vi "TTA_MATLAB_RFICPALLinearizationTest.vi"(0 "Sub-Function Name":string, 1 "Instrument Cluster In":T1, 5 "Test Group":string, 11 "error in":errorcluster) -> (4 "SubTestSuccess":dbl[](array[numeric]), 12 "Instrument Cluster Out":T1, 15 "error out":errorcluster)   [LabVIEW 2016]
uses:
  TTA_Controls/TTA_Control_Complete_Settings_Cluster.ctl
  TTA_Controls/TTA_Control_Instrument_Cluster.ctl
  TTA_Globals/TTA_Global_Complete_Settings.vi
panel:
  out "Test Status":string
  in  "Complete Settings Cluster":T2
  out "RFICs":i32[](array[numeric])
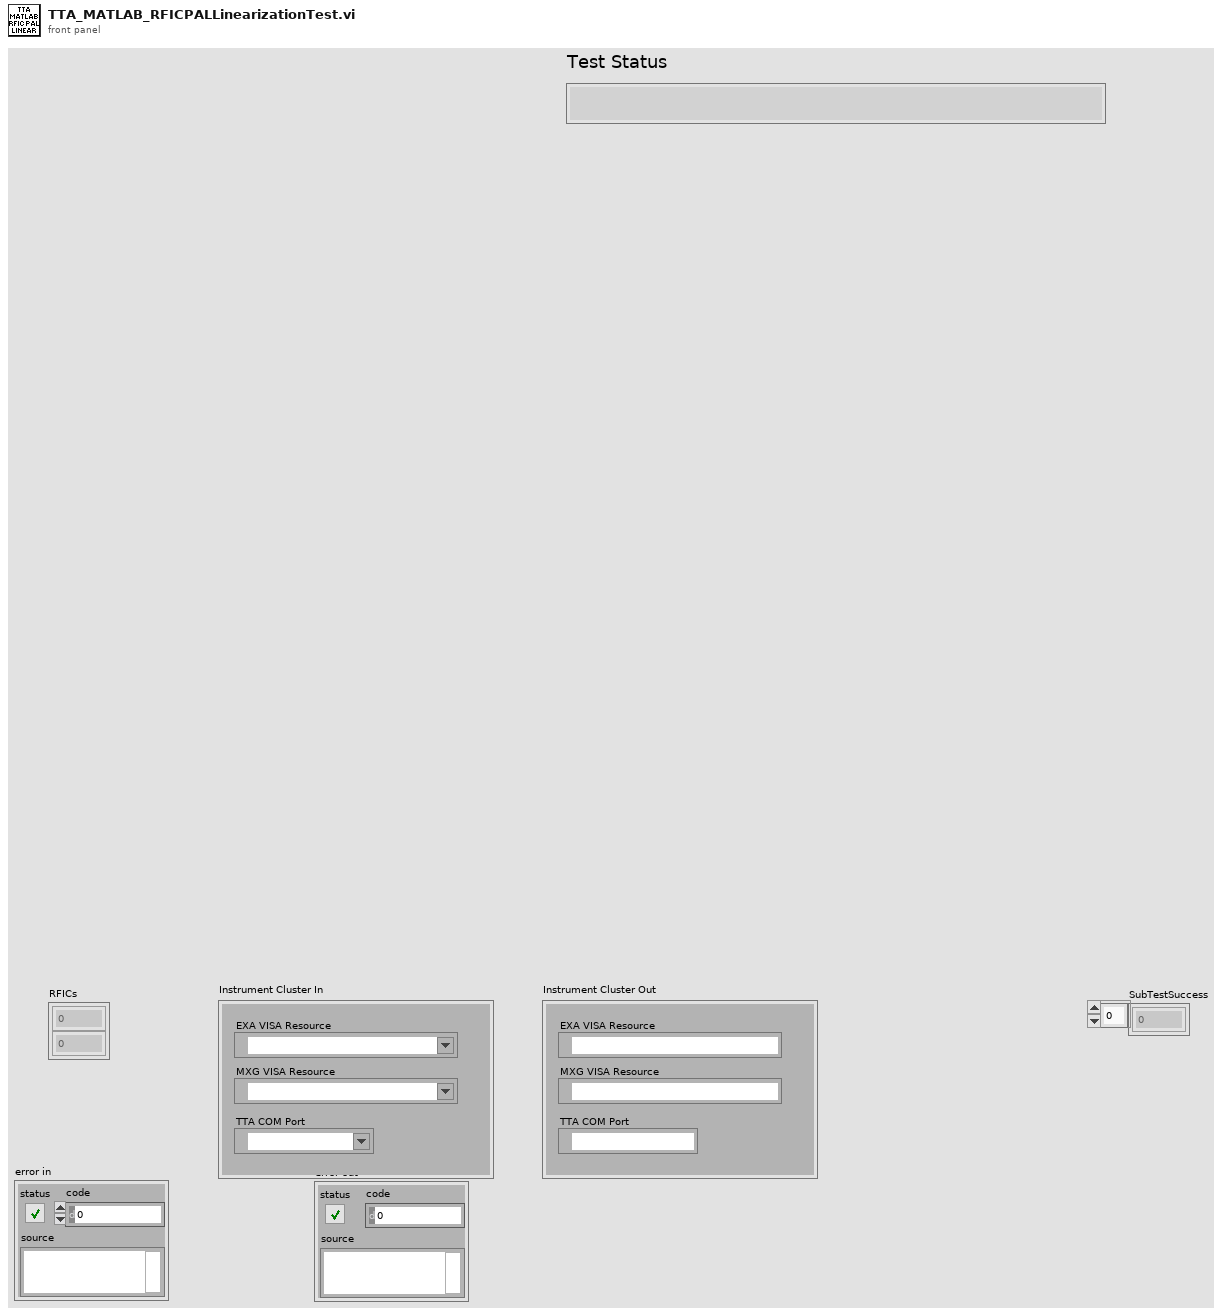
[diagram p1: front panel]
types:
  T1 = typedef "TTA_Control_Instrument_Cluster.ctl" = cluster{"EXA VISA Resource":refnum<visa-resource-name>, "MXG VISA Resource":refnum<visa-resource-name>, "TTA COM Port":refnum<visa-resource-name>}
  T2 = typedef "TTA_Control_Complete_Settings_Cluster.ctl" = cluster{"Brief Cluster":cluster{"STM Firmware File":string, "STM Firmware Address":string, "Required SW Version":string, "Template Used":string}, "Instrument Setting Cluster":cluster{"BDSFreq":dbl, "BDS Amp":dbl, "TxRFCal_Freq":dbl, "TxRFCal_Amp":dbl, "RxRFCal_Freq":dbl, "RxRFCal_Freq":dbl, "TxIF_Freq":dbl, "TxIF_Amp":dbl, "Tx_Output_Power_Signal_Freq":dbl, "Tx_ACPR_Signal_Freq":dbl, "Rx_RF_Freq":dbl, "Rx_RF_Amp":dbl, "Rx_Output_Power_Signal_Freq":dbl, "Rx_Output_Power_Sense_Freq":dbl}, "PAL Calibration\nInputs Cluster":cluster{"Amplitude Range\nMax(dBm)":dbl, "Amplitude Range\nMin(dBm)":dbl, "Amplitude Least\nCriteria (dBm)":dbl, "Frequency 1":dbl, "Frequency 2":dbl, "Frequency 3":dbl, "CAL Amplitude\nDecrement (dB)":dbl, "CAL Amplitude\nIncrement(dB)":dbl, "DownloadFile":string}, "TxOffset Cal Cluster":cluster{"Tx1 Offset (dB)":dbl, "Tx2 Offset (dB)":dbl, "Tx3 Offset (dB)":dbl, "Tx4 Offset (dB)":dbl, "Total RF Tx Loss (dB)":dbl}, "RxOffset Cal Cluster":cluster{"Rx1 Offset (dB)":dbl, "Rx2 Offset (dB)":dbl, "Rx3 Offset (dB)":dbl, "Rx4 Offset (dB)":dbl, "Total RF Rx Loss (dB)":dbl}, "TX Output Power Settings Cluster":cluster{"Frequency Sweep (MHz)":dbl[], "Sig Gen \nPower (dBm)":dbl, "Span (kHz)":dbl, "RBW (Hz)":dbl, "Ref Level (dBm)":dbl, "Low Power \nLimit":dbl, "High Power \nLimit":dbl, "DigAtt Max":dbl, "DigAtt Min":dbl}, "Tx ACPR Settings Cluster":cluster{"ACPR Filename":string, "Sampling Rate":dbl, "Power (dBm)":dbl, "IF Frequency Sweep (MHz)":dbl[], "State Name":string, "Mechanical\nAttenuation":dbl, "RefLevel Offset":dbl, "Amplitude Range\nMax (dBm)":dbl, "Amplitude Range\nMin (dBm)":dbl, "Cal Amp \nIncrement (dB)":dbl, "Cal Amp\nDecrement (dB)":dbl}, "Power Cal Cluster":cluster{"Power List (dBm)":dbl[], "Frequency (MHz)":dbl[], "Cal Decrement (dB)":dbl, "Cal Increment (dB)":dbl}, "Rx Received Power Settings Cluster":cluster{"Frequency Sweep (MHz)":dbl[], "Power (dBm)":dbl, "Span (kHz)":dbl, "RBW (Hz)":dbl, "Ref Level":dbl, "Low Power \nLimit (dBm)":dbl, "High Power\nLimit (dBm)":dbl}, "Tx Output Power Criteria Cluster":cluster{"CH1-TX1 \nMin":dbl, "CH1-TX1\nMax":dbl, "CH1-TXx3\nMin ":dbl, "CH1-TXx3\nMax":dbl, "CH2-TX1\nMin":dbl, "CH2-TX1\nMax":dbl, "CH2-TXx3\nMin":dbl, "CH2-TXx3\nMax":dbl}, "Tx ACPR Criteria Cluster":cluster{"Min Inband":dbl, "Max Close Outband":dbl, "Max Far Outband":dbl}, "Rx Output Power Criteria Cluster":cluster{"CH1-RX1 \nMin":dbl, "CH1-RX1 \nMax":dbl, "CH1-RXx3 \nMin":dbl, "CH1-RXx3\nMax":dbl, "CH2-RX1\nMin":dbl, "CH2-RX1\nMax":dbl, "CH2-RXx3\nMin":dbl, "CH2-RXx3\nMax":dbl}}
  T3 = cluster{"Amplitude Range\nMax(dBm)":dbl, "Amplitude Range\nMin(dBm)":dbl, "Amplitude Least\nCriteria (dBm)":dbl, "Frequency 1":dbl, "Frequency 2":dbl, "Frequency 3":dbl, "CAL Amplitude\nDecrement (dB)":dbl, "CAL Amplitude\nIncrement(dB)":dbl, "DownloadFile":string}
  T4 = cluster{"ACPR Filename":string, "Sampling Rate":dbl, "Power (dBm)":dbl, "IF Frequency Sweep (MHz)":dbl[], "State Name":string, "Mechanical\nAttenuation":dbl, "RefLevel Offset":dbl, "Amplitude Range\nMax (dBm)":dbl, "Amplitude Range\nMin (dBm)":dbl, "Cal Amp \nIncrement (dB)":dbl, "Cal Amp\nDecrement (dB)":dbl}
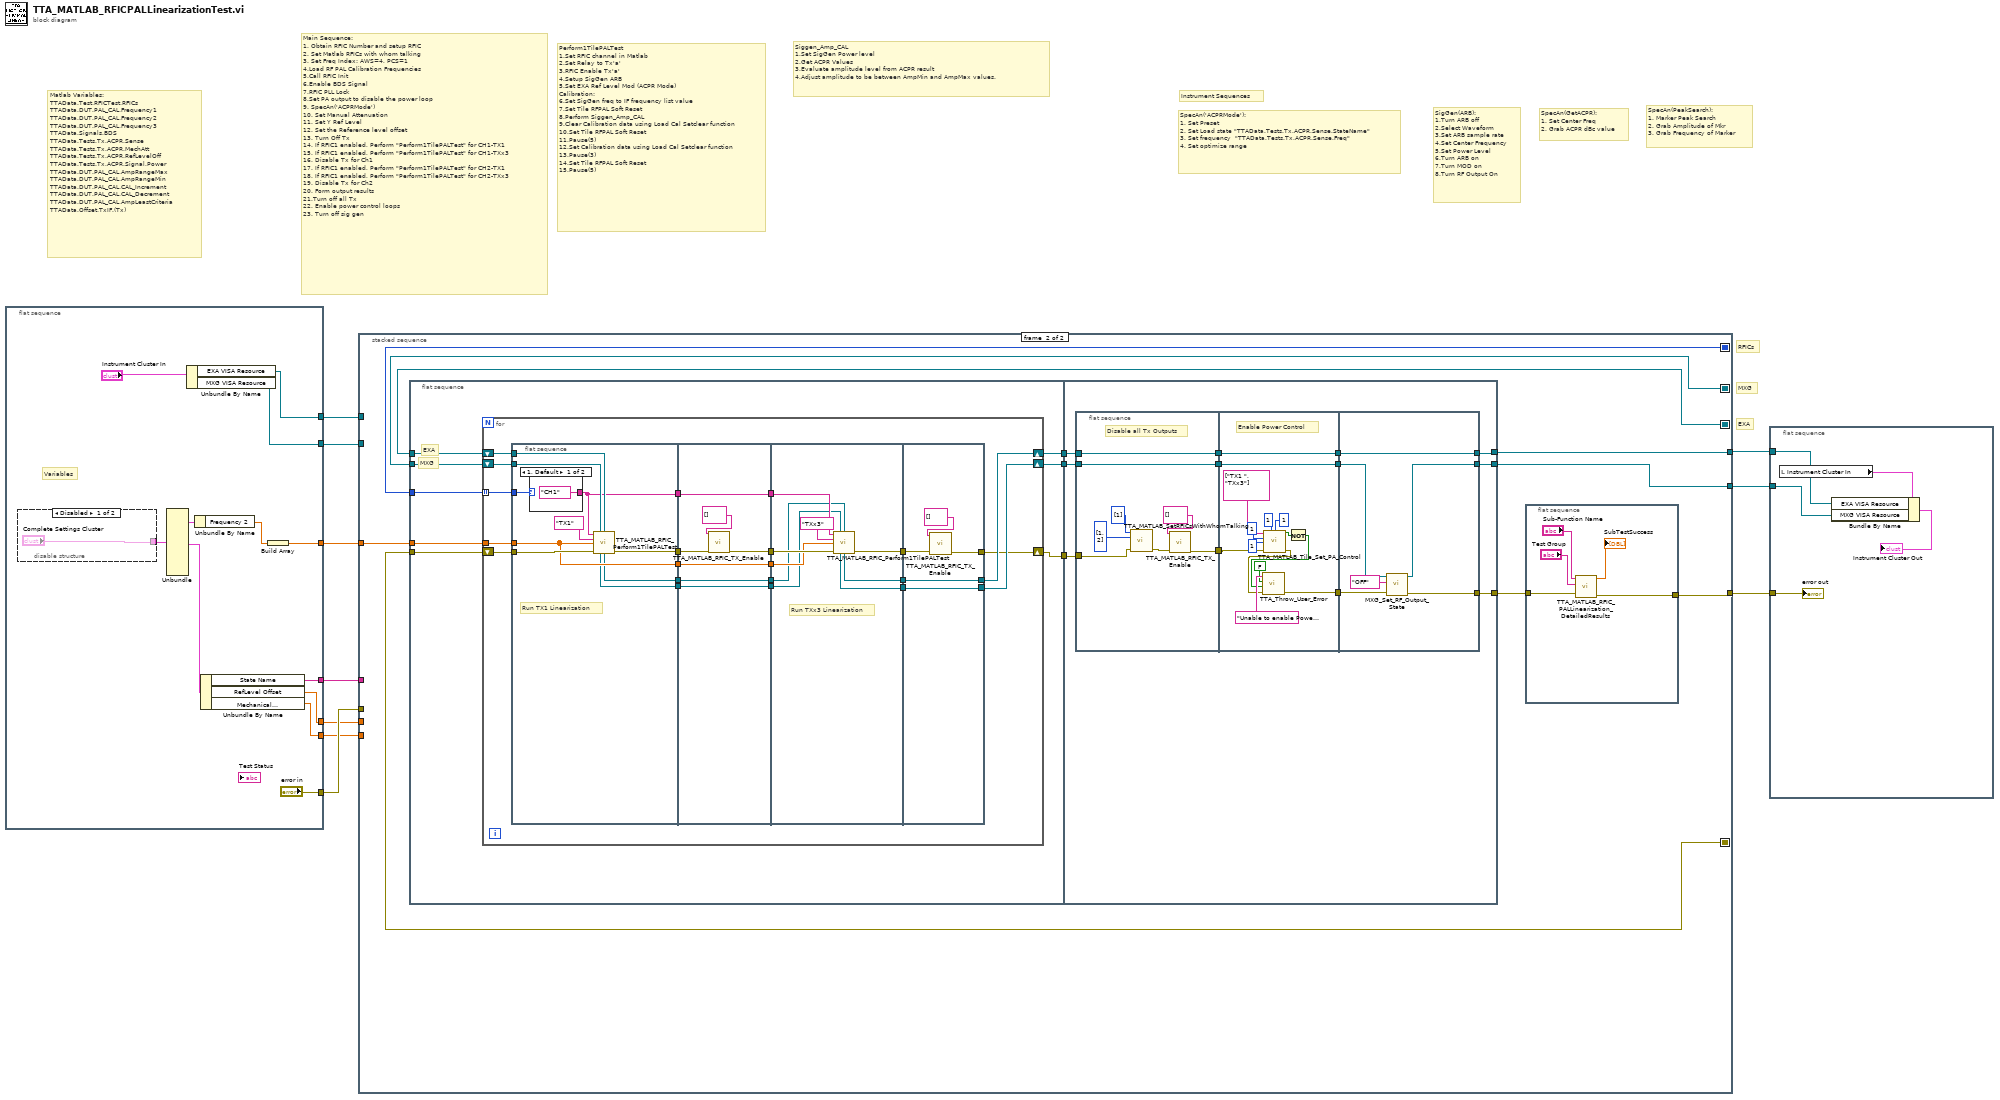
[diagram p0: block diagram]
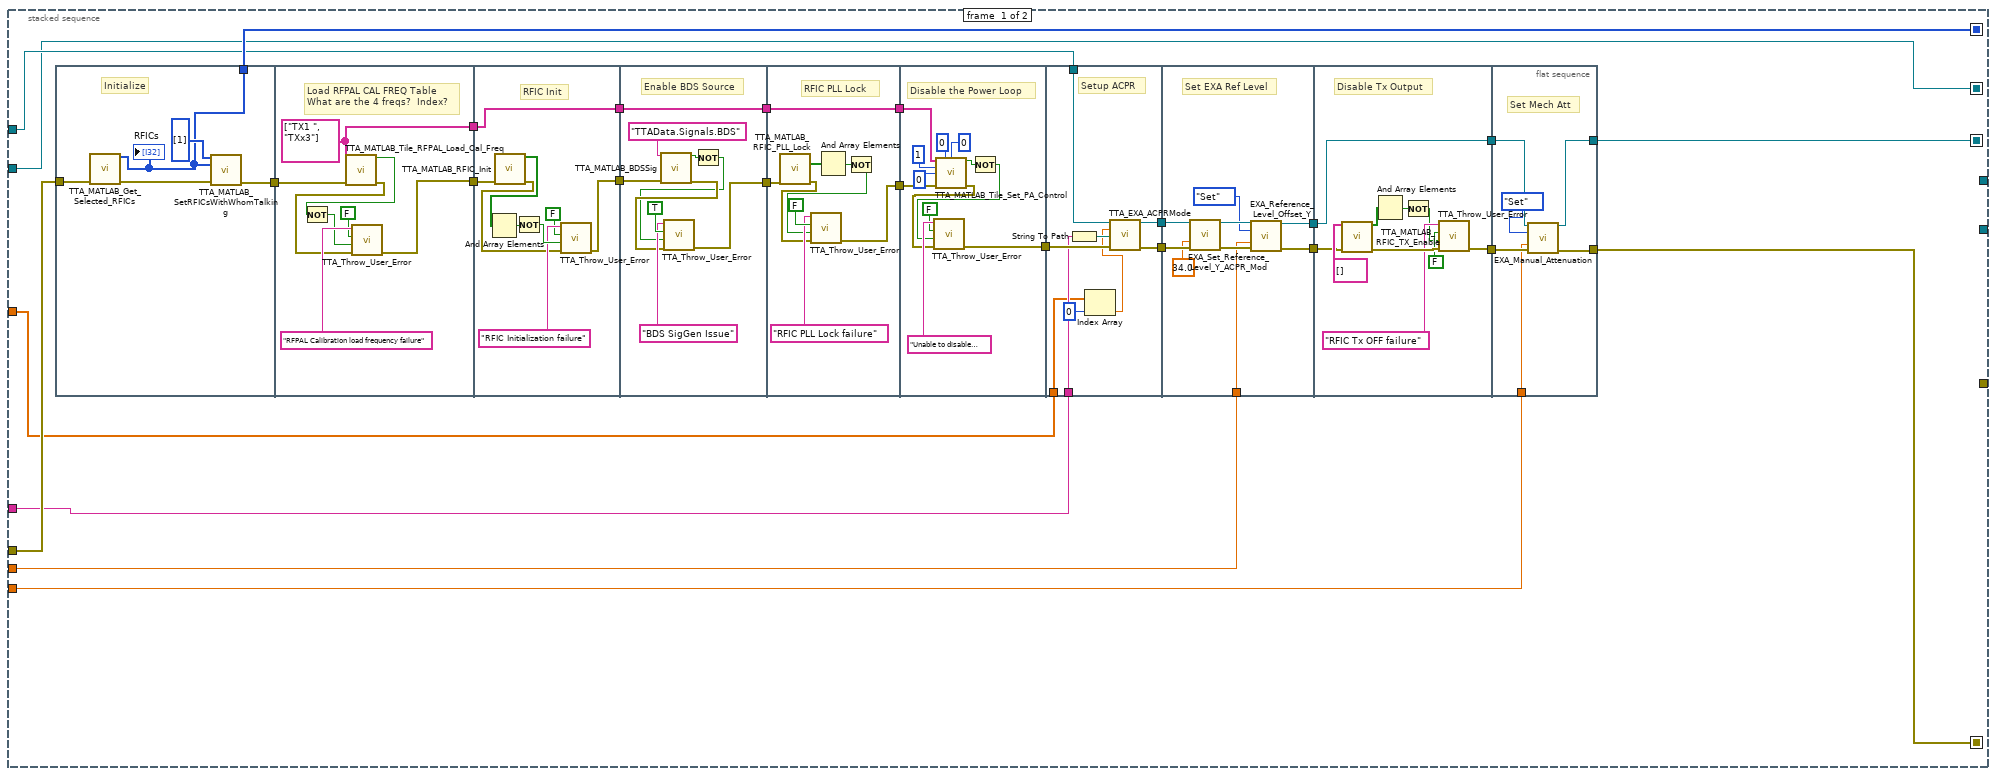
[diagram p2: hidden frame]
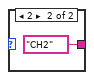
[diagram p3: hidden frame]
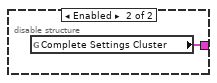
[diagram p4: hidden frame]
diagram:
  # "RFICs"
  # "EXA"
  # "MXG"
  # "SpecAn(GetACPR):\n1. Set Center Freq\n2. Grab ACPR dBc value"
  # "Siggen_Amp_CAL\n1.Set SigGen Power level\n2.Get ACPR Values \n3.Evaluate amplitude level from ACPR result\n4.Adjust amplitude to be between AmpMin and AmpMax values."
  # "Matlab Variables:\nTTAData.Test.RFICTest.RFICs\nTTAData.DUT.PAL_CAL.Frequency1\nTTAData.DUT.PAL_CAL.Frequency2\nTTAData.DUT.PAL_CAL.Frequency3\nTTAData.Signals.BDS\nTTAData.Tests.Tx.ACPR.Sense\nTTAData.Tests.Tx.ACPR.MechAtt\nTTAData.Tests.Tx.ACPR.RefLevelOff\nTTAData.Tests.Tx.ACPR.Signal.Power\nTTAData.DUT.PAL_CAL.AmpRangeMax\nTTAData.DUT.PAL_CAL.AmpRangeMin\nTTAData.DUT.PAL_CAL.CAL_Increment\nTTAData.DUT.PAL_CAL.CAL_Decrement\nTTAData.DUT.PAL_CAL.AmpLeastCriteria\nTTAData.Offset.TxIF.(Tx)"
  # "Instrument Sequences"
  # "SpecAn('ACPRMode'):\n1. Set Preset\n2. Set Load state \"TTAData.Tests.Tx.ACPR.Sense.StateName\"\n3. Set frequency  \"TTAData.Tests.Tx.ACPR.Sense.Freq\"\n4. Set optimize range"
  # "Main Sequence:\n1. Obtain RFIC Number and setup RFIC\n2. Set Matlab RFICs with whom talking\n3. Set Freq Index: AWS=4, PCS=1\n4.Load RF PAL Calibration Frequencies\n5.Call RFIC Init\n6.Enable BDS Signal\n7.RFIC PLL Lock\n8.Set PA output to disable the power loop\n9. SpecAn('ACPRMode')\n10. Set Manual Attenuation\n11. Set Y Ref Level\n12. Set the Reference level offset\n13. Turn Off Tx\n14. If RFIC1 enabled, Perform \"Perform1TilePALTest\" for CH1-TX1\n15. If RFIC1 enabled, Perform \"Perform1TilePALTest\" for CH1-TXx3\n16. Disable Tx for Ch1\n17. If RFIC1 enabled, Perform \"Perform1TilePALTest\" for CH2-TX1\n18. If RFIC1 enabled, Perform \"Perform1TilePALTest\" for CH2-TXx3\n19. Disable Tx for Ch2\n20. Form output results\n21.Turn off all Tx\n22. Enable power control loops\n23. Turn off sig gen"
  # "SpecAn(PeakSearch):\n1. Marker Peak Search\n2. Grab Amplitude of Mkr\n3. Grab Frequency of Marker"
  # "SigGen(ARB):\n1.Turn ARB off\n2.Select Waveform\n3.Set ARB sample rate\n4.Set Center Frequency\n5.Set Power Level\n6.Turn ARB on\n7.Turn MOD on\n8.Turn RF Output On"
  # "Perform1TilePALTest\n1.Set RFIC channel in Matlab\n2.Set Relay to Tx'a'\n3.RFIC Enable Tx'a'\n4.Setup SigGen ARB\n5.Set EXA Ref Level Mod (ACPR Mode)\nCalibration:\n6.Set SigGen freq to IF frequency list value\n7.Set Tile RFPAL Soft Reset\n8.Perform Siggen_Amp_CAL \n9.Clear Calibration data using Load Cal Setclear function\n10.Set Tile RFPAL Soft Reset\n11.Pause(5)\n12.Set Calibration data using Load Cal Setclear function\n13.Pause(3)\n14.Set Tile RFPAL Soft Reset\n15.Pause(5)"
  n1 = flat-sequence {
    tunnel: ["error in"] -> w10
    tunnel: [w13] -> w9
    tunnel: [w12] -> w8
    tunnel: [w20] -> w7
    tunnel: [w17] -> w6
    tunnel: [w18] -> w5
    tunnel: [w11] -> w1
    frame #0 {
      # "Variables"
      n2 = disable-structure shown="Disabled" {
        disable-tunnel: ["Complete Settings Cluster" w24] -> w22
        frame Disabled {
        }
        frame Enabled {
          n3 = global read "TTA_Global_Complete_Settings.vi" "Complete Settings Cluster"() -> (w24:T2)
        }
      }
      n4 = Unbundle(w22) -> ("PAL Calibration\nInputs Cluster"=w16:T3, "Tx ACPR Settings Cluster"=w19:T4)  [unwired: 10 out]
      n5 = Unbundle By Name("Instrument Cluster In") -> ("EXA VISA Resource"=w13:refnum<visa-resource-name>, "MXG VISA Resource"=w12:refnum<visa-resource-name>)
      n6 = Unbundle By Name(w16) -> ("Frequency 2"=w15:dbl)
      n7 = Unbundle By Name(w19) -> ("State Name"=w17:string, "RefLevel Offset"=w18:dbl, "Mechanical\nAttenuation"=w11:dbl)
      n8 = Build Array(w15) -> (w20:dbl[])
    }
  }
  n9 = stacked-sequence {
    seq-local: [w48 _] -> [_ w148]
    seq-local: [w47 _] -> [_ w146]
    seq-local: [w46 _] -> [_ w147]
    seq-local: [w28 _] -> [_ w144]
    tunnel: w10 -> [w50 _]
    tunnel: w9 -> [w34 _]
    tunnel: w8 -> [w28 _]
    tunnel: w7 -> [w35 w145]
    tunnel: w6 -> [w36 _]
    tunnel: w5 -> [w31 _]
    tunnel: [_ w137] -> w4
    tunnel: [_ w140] -> w3
    tunnel: [_ w139] -> w2
    tunnel: w1 -> [w25 _]
    frame #0 {
      n10 = flat-sequence {
        tunnel: w50 -> [w53]
        tunnel: [w52] -> w48
        tunnel: [w51] -> w45
        tunnel: w45 -> [w63]
        tunnel: [w57] -> w44
        tunnel: [w56] -> w41
        tunnel: w44 -> [w67]
        tunnel: [w65] -> w43
        tunnel: w41 -> [w64]
        tunnel: [w64] -> w40
        tunnel: w43 -> [w77]
        tunnel: [w75] -> w42
        tunnel: w40 -> [w73]
        tunnel: [w73] -> w39
        tunnel: [w87] -> w49
        tunnel: w42 -> [w84]
        tunnel: w39 -> [w82]
        tunnel: [w82] -> w38
        tunnel: w49 -> [w98]
        tunnel: [w93] -> w37
        tunnel: w38 -> [w92]
        tunnel: w37 -> [w111]
        tunnel: w36 -> [w109]
        tunnel: w35 -> [w105]
        tunnel: w34 -> [w108]
        tunnel: [w107] -> w33
        tunnel: [w106] -> w32
        tunnel: w33 -> [w119]
        tunnel: w32 -> [w120]
        tunnel: w31 -> [w115]
        tunnel: [w113] -> w30
        tunnel: [w112] -> w29
        tunnel: w30 -> [w122]
        tunnel: w29 -> [w121]
        tunnel: [w121] -> w27
        tunnel: [w123] -> w26
        tunnel: [w135] -> w47
        tunnel: [w133] -> w46
        tunnel: w27 -> [w134]
        tunnel: w26 -> [w136]
        tunnel: w25 -> [w131]
        frame #0 {
          # "Initialize"
          n11 = call "TTA_MATLAB_Get_Selected_RFICs.vi"("error in"=w53) -> ("RFICs"=w52:i32[], "error out"=w54:errorcluster)  [unwired: 13 in]
          "RFICs" <- w52
          n12 = call "TTA_MATLAB_SetRFICsWithWhomTalking.vi"("Panel Array"=i32[] [1], "RFIC Array"=w52, "error in"=w54) -> ("error out"=w51:errorcluster)  [unwired: 12 in]
        }
        frame #1 {
          w56 = string[] ["TX1 ", "TXx3"] ("Channels")
          # "Load RFPAL CAL FREQ Table\nWhat are the 4 freqs?  Index?"
          n13 = call "TTA_MATLAB_Tile_RFPAL_Load_Cal_Freq.vi"("Channels"=w56, "error in"=w63) -> ("Success"=w60:bool, "error out"=w58:errorcluster)  [unwired: 11 in, 1 out]
          n14 = Not(x=w60) -> (.not. x?=w59:bool)
          n15 = call "TTA_Throw_User_Error.vi"("error in"=w58, "Error?"=w59, "Stop Execution on Fail"=FALSE, "Error Message"="RFPAL Calibration load frequency failure") -> ("error out"=w57:errorcluster)  [unwired: 7 in]
        }
        frame #2 {
          # "RFIC Init"
          n16 = call "TTA_MATLAB_RFIC_Init.vi"("error in"=w67) -> ("SuccessComm"=w72:bool[], "error out"=w66:errorcluster)  [unwired: 13 in]
          n17 = And Array Elements(Boolean array=w72) -> (logical AND=w71:bool)
          n18 = Not(x=w71) -> (.not. x?=w70:bool)
          n19 = call "TTA_Throw_User_Error.vi"("error in"=w66, "Error?"=w70, "Stop Execution on Fail"=FALSE, "Error Message"="RFIC Initialization failure") -> ("error out"=w65:errorcluster)  [unwired: 7 in]
        }
        frame #3 {
          # "Enable BDS Source"
          n20 = call "TTA_MATLAB_BDSSig.vi"("Signal Settings"="TTAData.Signals.BDS", "error in"=w77) -> ("Success"=w78:bool, "error out"=w76:errorcluster)  [unwired: 12 in]
          n21 = Not(x=w78) -> (.not. x?=w74:bool)
          n22 = call "TTA_Throw_User_Error.vi"("error in"=w76, "Error?"=w74, "Stop Execution on Fail"=TRUE, "Error Message"="BDS SigGen Issue") -> ("error out"=w75:errorcluster)  [unwired: 7 in]
        }
        frame #4 {
          # "RFIC PLL Lock"
          n23 = call "TTA_MATLAB_RFIC_PLL_Lock.vi"("error in"=w84) -> ("SuccessComm"=w90:bool[], "error out"=w83:errorcluster)  [unwired: 11 in, 2 out]
          n24 = And Array Elements(Boolean array=w90) -> (logical AND=w86:bool)
          n25 = Not(x=w86) -> (.not. x?=w85:bool)
          n26 = call "TTA_Throw_User_Error.vi"("error in"=w83, "Error?"=w85, "Stop Execution on Fail"=FALSE, "Error Message"="RFIC PLL Lock failure") -> ("error out"=w87:errorcluster)  [unwired: 7 in]
        }
        frame #5 {
          # "Disable the Power Loop"
          n27 = call "TTA_MATLAB_Tile_Set_PA_Control.vi"("Channels"=w92, "OutPower"=0, "InPower"=0, "Temp"=1, "Current"=0, "error in"=w98) -> ("Success"=w95:bool, "error out"=w91:errorcluster)  [unwired: 6 in, 2 out]
          n28 = Not(x=w95) -> (.not. x?=w94:bool)
          n29 = call "TTA_Throw_User_Error.vi"("error in"=w91, "Error?"=w94, "Stop Execution on Fail"=FALSE, "Error Message"="Unable to disable Power Loop") -> ("error out"=w93:errorcluster)  [unwired: 7 in]
        }
        frame #6 {
          # "Setup ACPR"
          n30 = String To Path(string=w109) -> (path=w110:path)
          n31 = Index Array(array=w105, index=0) -> (element=w103:dbl)
          n32 = call "TTA_EXA_ACPRMode.vi"("VISA resource In"=w108, "Frequency (MHz)"=w103, "State File"=w110, "error in"=w111) -> ("VISA resource Out"=w107:refnum<visa-resource-name>, "error out"=w106:errorcluster)  [unwired: 10 in]
        }
        frame #7 {
          # "Set EXA Ref Level"
          n33 = call "EXA_Set_Reference_Level_Y_ACPR_Mod.vi"("VISA resource name"=w119, "Reference Level \nOffset (dBm)"=34.0 ("Reference Level \nOffset (dBm)"), "error in"=w120) -> ("VISA resource name"=w116:refnum<visa-resource-name>, "error out"=w117:errorcluster)  [unwired: 11 in]
          n34 = call "EXA_Reference_Level_Offset_Y.vi"("VISA resource name"=w116, "Mode"=enum16{"Set", "Get"}."Set", "Reference Level \nOffset (dBm)"=w115, "error in"=w117) -> ("VISA resource name"=w112:refnum<visa-resource-name>, "error out"=w113:errorcluster)  [unwired: 9 in, 1 out]
        }
        frame #8 {
          # "Disable Tx Output"
          n35 = call "TTA_MATLAB_RFIC_TX_Enable.vi"("Channels"=string[] [], "error in"=w122) -> ("SuccessComm"=w125:bool[], "error out"=w129:errorcluster)  [unwired: 12 in]
          n36 = And Array Elements(Boolean array=w125) -> (logical AND=w126:bool)
          n37 = Not(x=w126) -> (.not. x?=w124:bool)
          n38 = call "TTA_Throw_User_Error.vi"("error in"=w129, "Error?"=w124, "Stop Execution on Fail"=FALSE, "Error Message"="RFIC Tx OFF failure") -> ("error out"=w123:errorcluster)  [unwired: 7 in]
        }
        frame #9 {
          # "Set Mech Att"
          n39 = call "EXA_Manual_Attenuation.vi"("VISA resource name"=w134, "Mode"=enum16{"Set", "Get"}."Set", "Attenuation (dB)"=w131, "error in"=w136) -> ("VISA resource name"=w133:refnum<visa-resource-name>, "error out"=w135:errorcluster)  [unwired: 9 in, 1 out]
        }
      }
    }
    frame #1 {
      n40 = flat-sequence {
        tunnel: w148 -> [w161]
        tunnel: w147 -> [w160]
        tunnel: w144 -> [w159]
        tunnel: w146 -> [w158]
        tunnel: w145 -> [w157]
        tunnel: [w156] -> w143
        tunnel: [w155] -> w142
        tunnel: [w154] -> w141
        tunnel: w143 -> [w227]
        tunnel: w142 -> [w226]
        tunnel: w141 -> [w225]
        tunnel: [w218] -> w138
        tunnel: [w217] -> w140
        tunnel: [w216] -> w139
        frame #0 {
          # "EXA"
          # "MXG"
          n41 = for {
            tunnel: w161 -> [w182] mode=indexing
            tunnel: w157 -> [w178]
            shift-right: [w177] -> w155
            shift-left: w160 -> [w181]
            shift-right: [w176] -> w154
            shift-left: w159 -> [w180]
            shift-right: [w162] -> w156
            shift-left: w158 -> [w179]
            n42 = flat-sequence {
              tunnel: w182 -> [w192]
              tunnel: w181 -> [w190]
              tunnel: w180 -> [w189]
              tunnel: w179 -> [w188]
              tunnel: [w187] -> w172
              tunnel: [w186] -> w170
              tunnel: w178 -> [w185]
              tunnel: [w185] -> w168
              tunnel: [w184] -> w166
              tunnel: [w183] -> w164
              tunnel: w172 -> [w201]
              tunnel: [w201] -> w171
              tunnel: w170 -> [w196]
              tunnel: [w195] -> w169
              tunnel: w168 -> [w200]
              tunnel: [w200] -> w167
              tunnel: w166 -> [w199]
              tunnel: [w199] -> w165
              tunnel: w164 -> [w198]
              tunnel: [w198] -> w163
              tunnel: w171 -> [w209]
              tunnel: w169 -> [w208]
              tunnel: w167 -> [w207]
              tunnel: w165 -> [w205]
              tunnel: w163 -> [w204]
              tunnel: [w206] -> w175
              tunnel: [w203] -> w174
              tunnel: [w202] -> w173
              tunnel: [w214] -> w177
              tunnel: [w215] -> w176
              tunnel: w175 -> [w212]
              tunnel: w174 -> [w215]
              tunnel: w173 -> [w214]
              tunnel: [w211] -> w162
              frame #0 {
                # "Run TX1 Linearization"
                n43 = case shown="1, Default" w192 {
                  tunnel: ["CH1" ("Channel") "CH2" ("Channel")] -> w187
                  frame 1, Default {
                  }
                  frame 2 {
                  }
                }
                n44 = call "TTA_MATLAB_RFIC_Perform1TilePALTest.vi"("Channel"=w187, "MXG VISA Resource In"=w189, "EXA VISA Resource"=w190, "Tx"="TX1", "Freq_Cal_List"=w185, "error in"=w188) -> ("MXG VISA Resource Out"=w184:refnum<visa-resource-name>, "EXA VISA Resource Out"=w183:refnum<visa-resource-name>, "error out"=w186:errorcluster)  [unwired: 7 in]
              }
              frame #1 {
                n45 = call "TTA_MATLAB_RFIC_TX_Enable.vi"("Channels"=string[] [], "error in"=w196) -> ("error out"=w195:errorcluster)  [unwired: 12 in, 1 out]
              }
              frame #2 {
                # "Run TXx3 Linearization"
                n46 = call "TTA_MATLAB_RFIC_Perform1TilePALTest.vi"("Channel"=w209, "MXG VISA Resource In"=w205, "EXA VISA Resource"=w204, "Tx"="TXx3", "Freq_Cal_List"=w207, "error in"=w208) -> ("MXG VISA Resource Out"=w203:refnum<visa-resource-name>, "EXA VISA Resource Out"=w202:refnum<visa-resource-name>, "error out"=w206:errorcluster)  [unwired: 7 in]
              }
              frame #3 {
                n47 = call "TTA_MATLAB_RFIC_TX_Enable.vi"("Channels"=string[] [], "error in"=w212) -> ("error out"=w211:errorcluster)  [unwired: 12 in, 1 out]
              }
            }
          }
        }
        frame #1 {
          n48 = flat-sequence {
            tunnel: w227 -> [w233]
            tunnel: w226 -> [w229]
            tunnel: w225 -> [w228]
            tunnel: [w230] -> w224
            tunnel: [w229] -> w223
            tunnel: [w228] -> w222
            tunnel: w224 -> [w238]
            tunnel: w223 -> [w249]
            tunnel: w222 -> [w248]
            tunnel: [w249] -> w221
            tunnel: [w248] -> w220
            tunnel: [w236] -> w219
            tunnel: [w252] -> w217
            tunnel: [w255] -> w216
            tunnel: w221 -> [w255]
            tunnel: w220 -> [w253]
            tunnel: w219 -> [w254]
            tunnel: [w250] -> w218
            frame #0 {
              # "Disable all Tx Outputs"
              n49 = call "TTA_MATLAB_SetRFICsWithWhomTalking.vi"("Panel Array"=i32[] [1], "RFIC Array"=i32[] [1, 2], "error in"=w233) -> ("error out"=w231:errorcluster)  [unwired: 12 in]
              n50 = call "TTA_MATLAB_RFIC_TX_Enable.vi"("Channels"=string[] [], "error in"=w231) -> ("error out"=w230:errorcluster)  [unwired: 12 in, 1 out]
            }
            frame #1 {
              # "Enable Power Control"
              n51 = call "TTA_MATLAB_Tile_Set_PA_Control.vi"("Channels"=string[] ["TX1 ", "TXx3"], "OutPower"=1, "InPower"=1, "Temp"=1, "Current"=1, "error in"=w238) -> ("Success"=w241:bool, "error out"=w239:errorcluster)  [unwired: 6 in, 2 out]
              n52 = Not(x=w241) -> (.not. x?=w240:bool)
              n53 = call "TTA_Throw_User_Error.vi"("error in"=w239, "Error?"=w240, "Stop Execution on Fail"=FALSE, "Error Message"="Unable to enable Power Loop") -> ("error out"=w236:errorcluster)  [unwired: 7 in]
            }
            frame #2 {
              n54 = call "MXG_Set_RF_Output_State.vi"("error in"=w254, "RF Output State"="OFF", "VISA resource name"=w253) -> ("error out"=w250:errorcluster, "VISA resource name"=w252:refnum<visa-resource-name>)  [unwired: 7 in]
            }
          }
        }
      }
      n55 = flat-sequence {
        tunnel: w138 -> [w153]
        tunnel: [w152] -> w137
        frame #0 {
          n56 = call "TTA_MATLAB_RFIC_PALLinearization_DetailedResults.vi"("error in"=w153, "TestGroup"="Test Group", "SubTest"="Sub-Function Name") -> ("error out"=w152:errorcluster, "SubTestSuccess"=→"SubTestSuccess":dbl[])  [unwired: 7 in]
        }
      }
    }
  }
  n57 = flat-sequence {
    tunnel: w4 -> [w260]
    tunnel: w3 -> [w257]
    tunnel: w2 -> [w258]
    frame #0 {
      n58 = local read "Instrument Cluster In"() -> (w256:T1)
      n59 = Bundle By Name(cluster=w256, "EXA VISA Resource"=w258, "MXG VISA Resource"=w257) -> (→"Instrument Cluster Out":T1)
      "error out" <- w260
    }
  }
